vi "LaserSetPower.vi"(7 "error in (no error)":errorcluster, 9 "Power":dbl, 10 "reference In":refnum<k24>) -> (0 "error out":errorcluster, 3 "reference out":refnum<k24>)   [LabVIEW 2019]
doc: "Generates sample waveforms according to the signal type in the HW Config input."
uses:
  E:/DevHardSoftware/MMicroscopy/HardwareAdapter/Lasers/Dependencies/Oxxius_Boxx.dll
  Dependencies/Oxxius_Boxx.dll
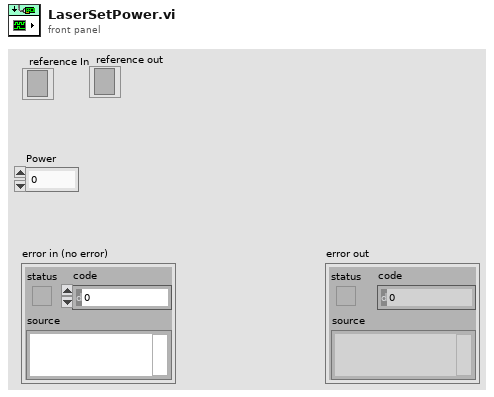
[diagram p1: front panel]
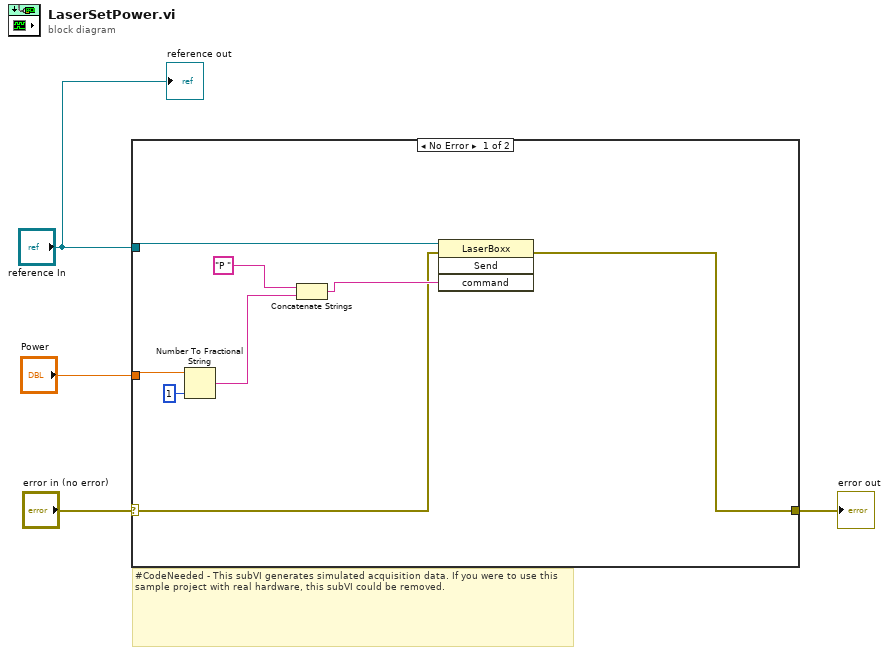
[diagram p0: block diagram]
diagram:
  # "#CodeNeeded - This subVI generates simulated acquisition data. If you were to use this sample project with real hardware, this subVI could be removed."
  n1 = case shown="No Error" "error in (no error)" {
    selector: "error in (no error)" -> [w5 w13]
    tunnel: [w11 w13] -> w3
    tunnel: "Power" -> [w10 _]
    tunnel: "reference In" -> [w12 _]
    frame No Error {
      n2 = Number To Fractional String(number=w10, precision (6)=i16 1) -> (F-format string=w7:string)  [unwired: 2 in]
      n3 = Concatenate Strings("P " ("command"), w7) -> (w6:string)
      n4 = invoke class="LaserBoxx" method="Send"(reference=w12, error in=w5, "command"=w6) -> (error out=w11:errorcluster)  [unwired: 1 in, 3 out]
    }
    frame Error {
    }
  }
  "error out" <- w3
  "reference out" <- "reference In"
